vi "Chart.vi"() -> ()   [LabVIEW 2020]
uses:
  <userlib>/_NEVSTOP/Communicable State Machine(CSM)/AdvanceAPI/CSM - Revert Arguments-Safe String.vi
  <userlib>/_NEVSTOP/Communicable State Machine(CSM)/_Shared/Trim Single-line Text.vi
  <userlib>/_NEVSTOP/Communicable State Machine(CSM)/AdvanceAPI/CSM - Make String Arguments Safe.vi
  <userlib>/_NEVSTOP/Communicable State Machine(CSM)/AdvanceAPI/CSM - Break Down Multiple States String.vi
  <userlib>/_NEVSTOP/Communicable State Machine(CSM)/AdvanceAPI/CSM - Compact Multiple States.vi
  <userlib>/_NEVSTOP/Communicable State Machine(CSM)/AdvanceAPI/CSM - Keywords.vi
  <userlib>/_NEVSTOP/Communicable State Machine(CSM)/Communicable State Machine.lvlib
panel:
  out "Waveform Chart":dbl(graph)
  out "State History":string
  in  "Name (\"\" to Use UUID)":string="Event CSM"
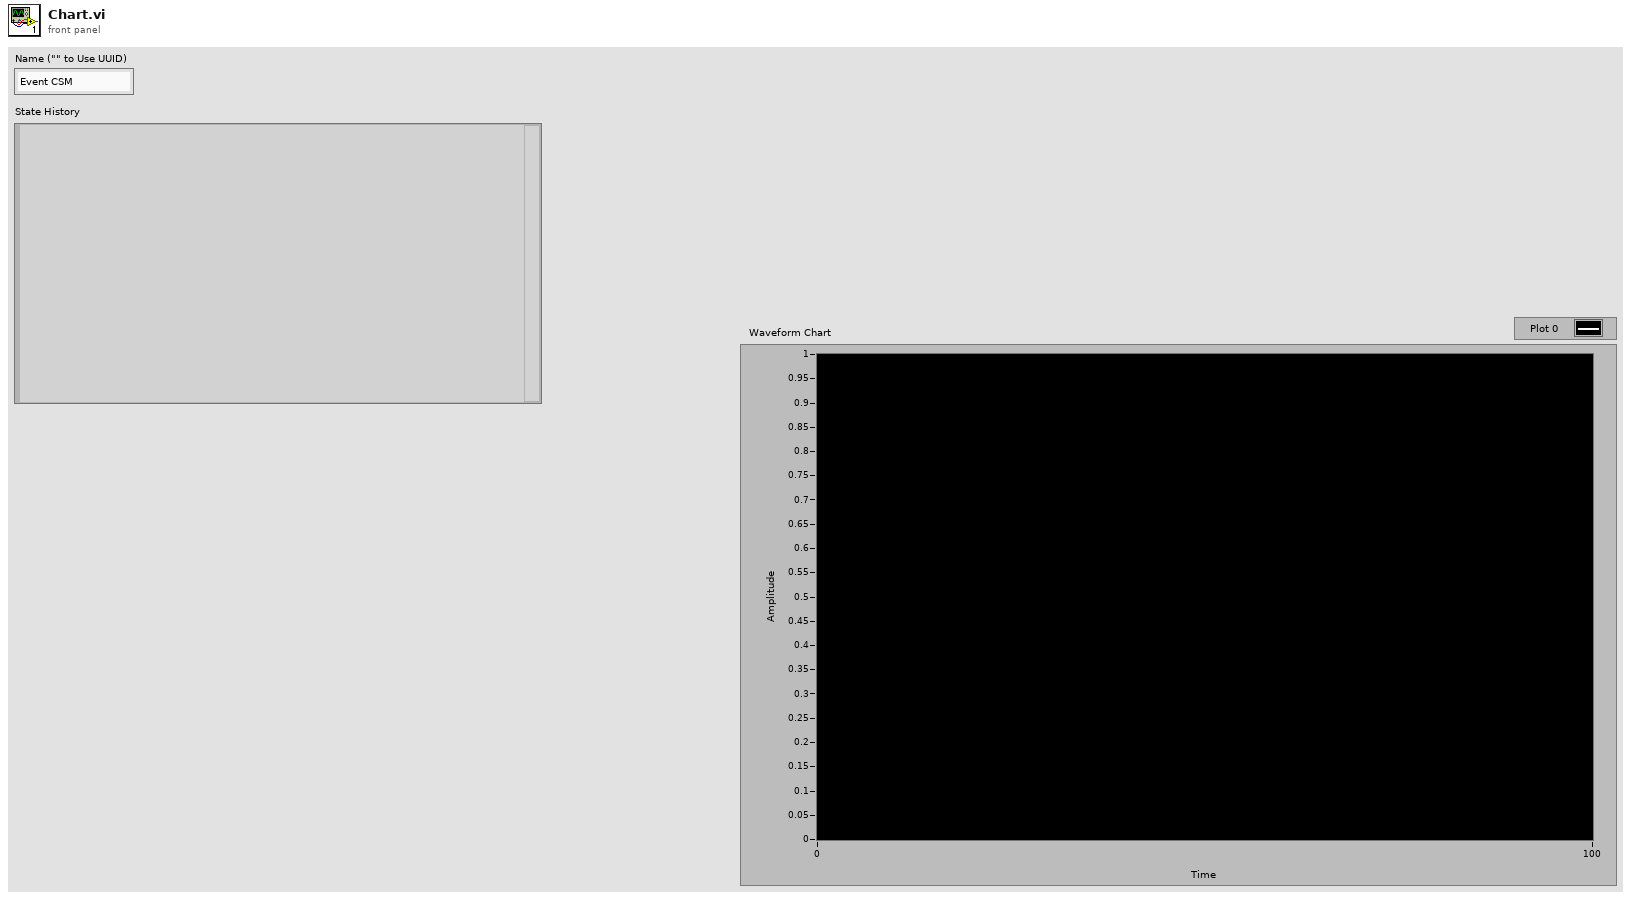
[diagram p1: front panel]
types:
  T1 = enum32{"Invalid", "Standard", "Closed", "Hidden", "Minimized", "Maximized"}
  T2 = enum32{"invalid app kind", "Development System", "Run Time System", "Student Edition", "Embedded LabVIEW", "Evaluation", "Custom"}
  T3 = typedef "Communicable State Machine.lvlib/_CSM_Response Source Message.ctl" = cluster{"‘State":string, "’Arguments":string, "’Error":errorcluster}
  T4 = cluster{"Current VI Reference":refnum<vi>, "Close Panel on Exit?":bool}
  T5 = cluster{"Core":cluster{"Current VI Reference":refnum<vi>, "Close Panel on Exit?":bool}, "Your Boolean data":bool, "Your string data":string}
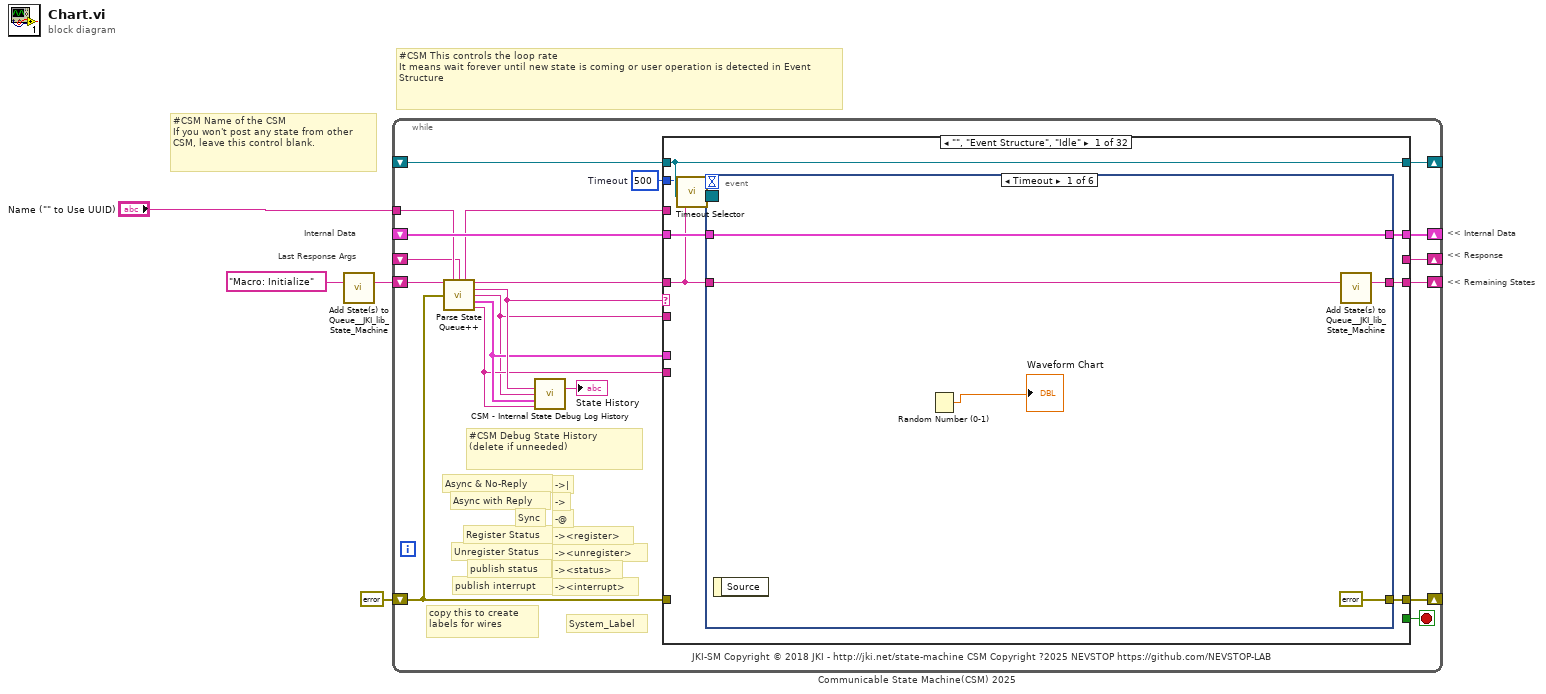
[diagram p0: block diagram]
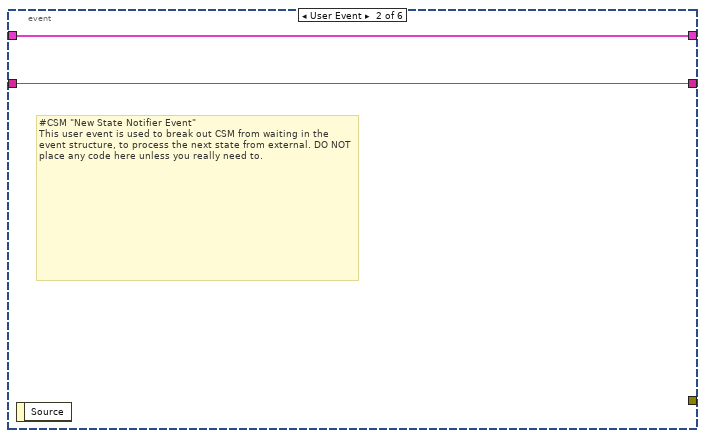
[diagram p2: hidden frame]
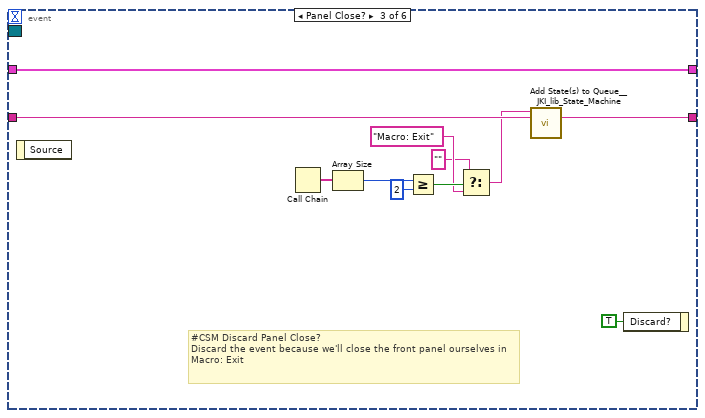
[diagram p3: hidden frame]
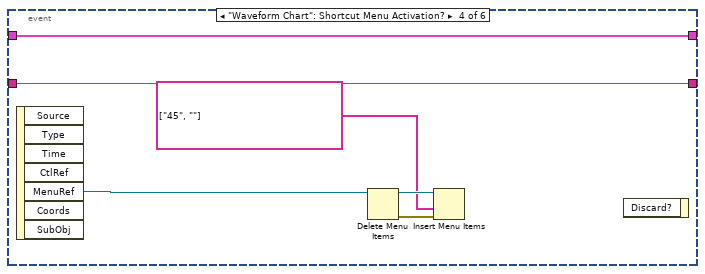
[diagram p4: hidden frame]
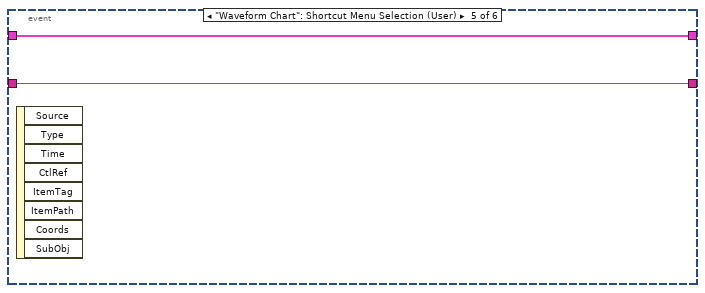
[diagram p5: hidden frame]
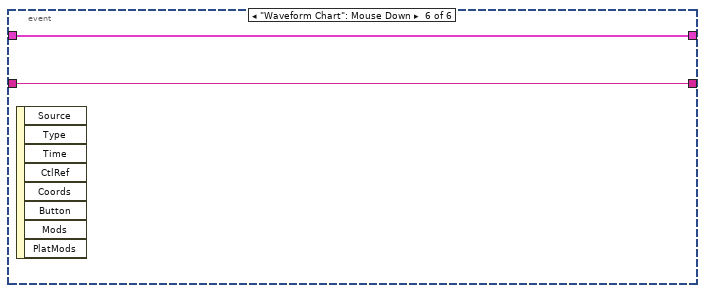
[diagram p6: hidden frame]
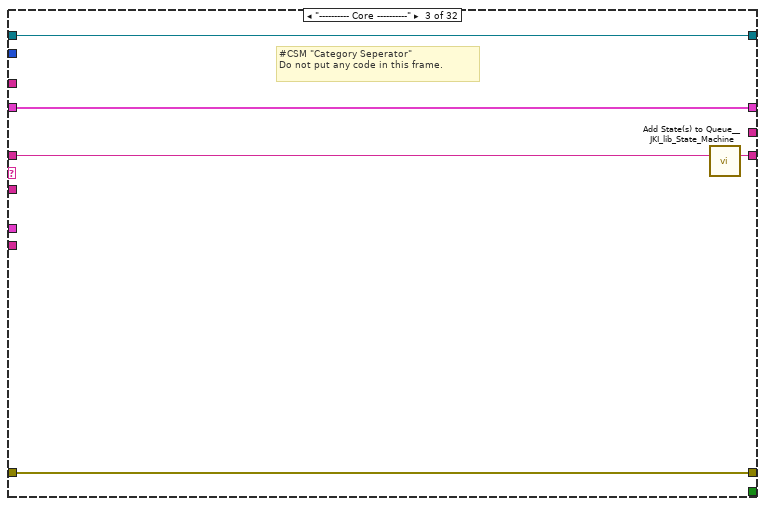
[diagram p8: hidden frame]
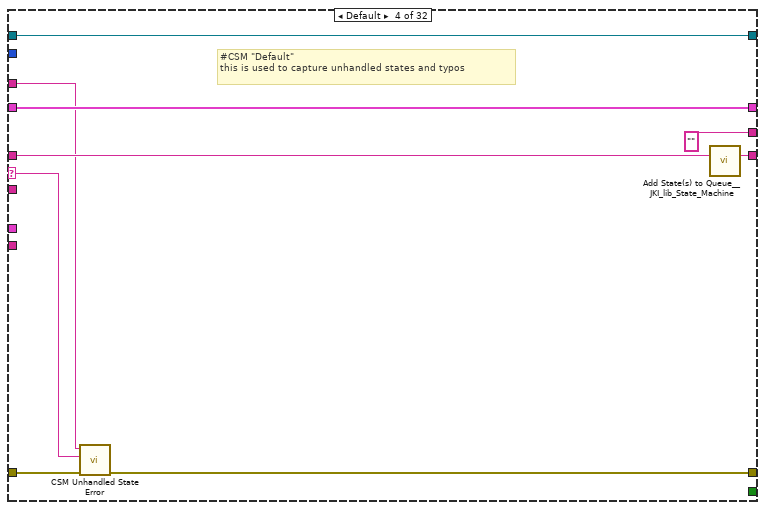
[diagram p9: hidden frame]
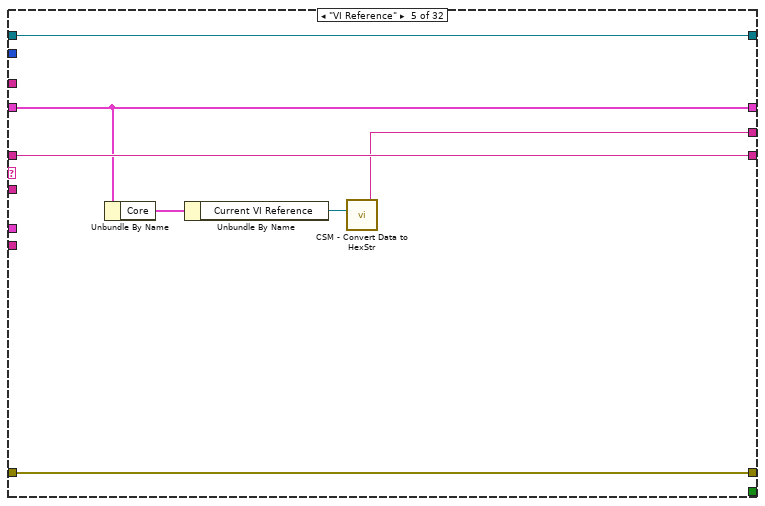
[diagram p10: hidden frame]
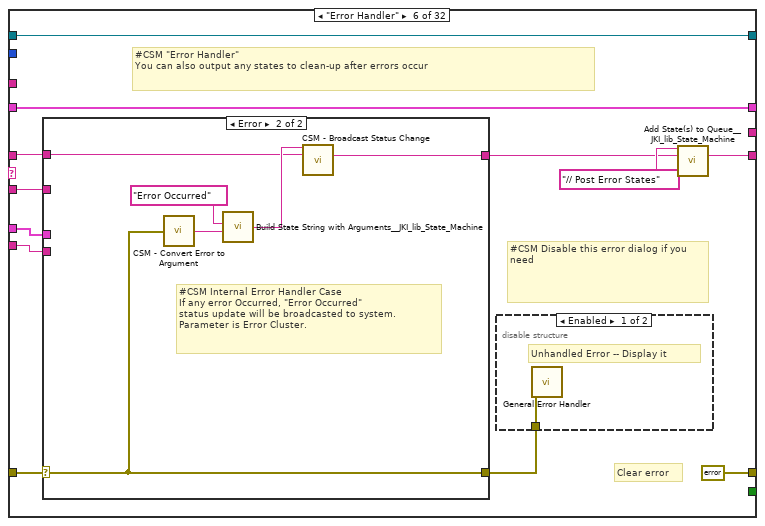
[diagram p11: hidden frame]
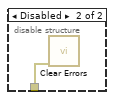
[diagram p12: hidden frame]
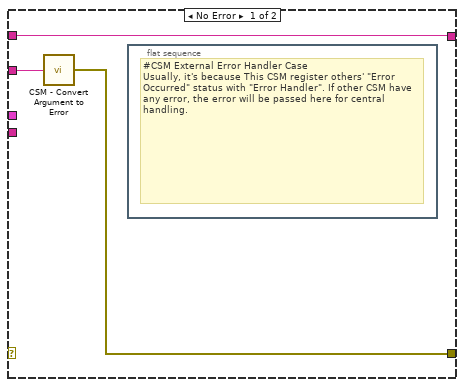
[diagram p13: hidden frame]
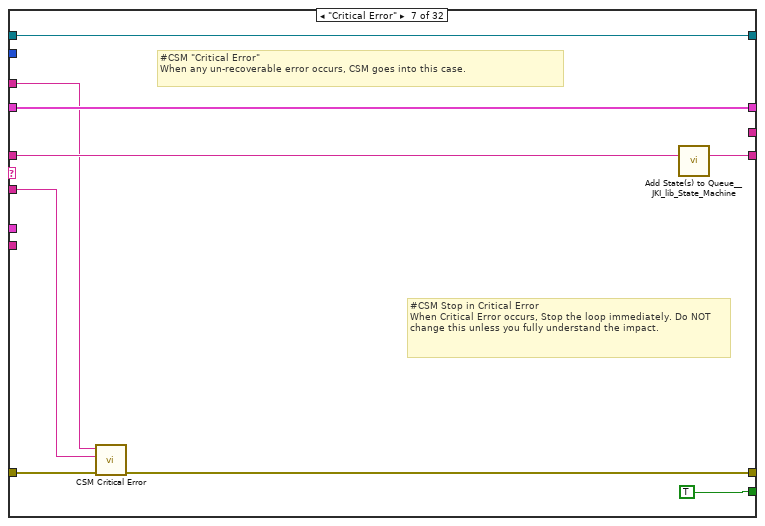
[diagram p14: hidden frame]
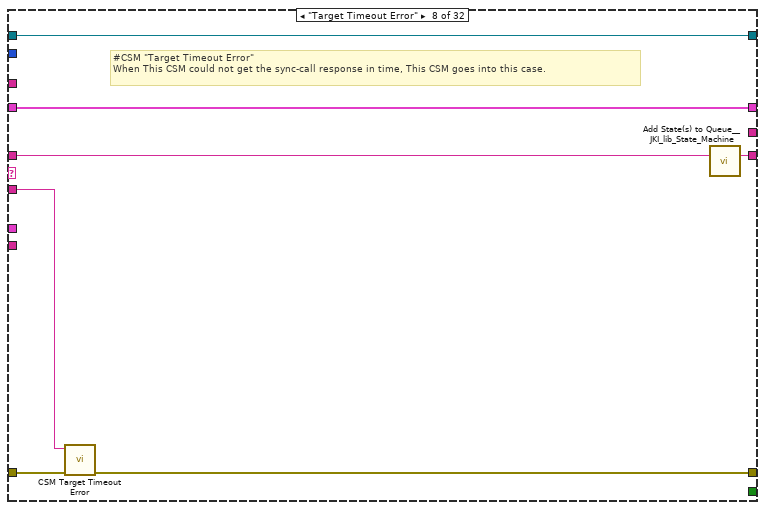
[diagram p15: hidden frame]
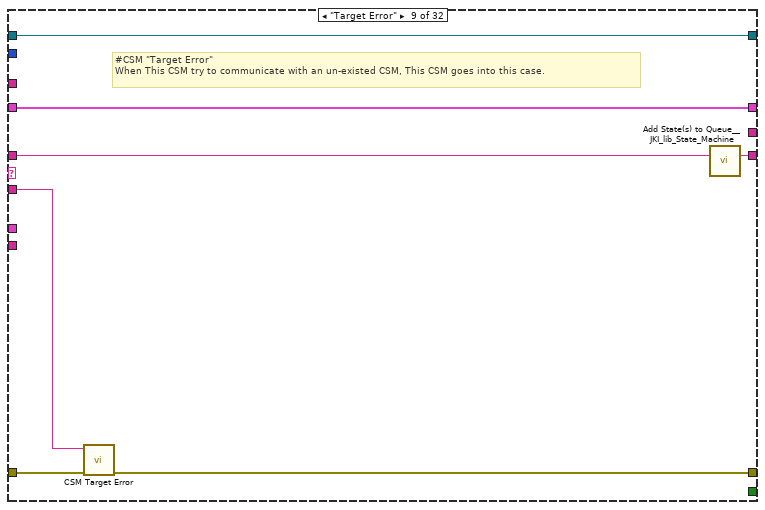
[diagram p16: hidden frame]
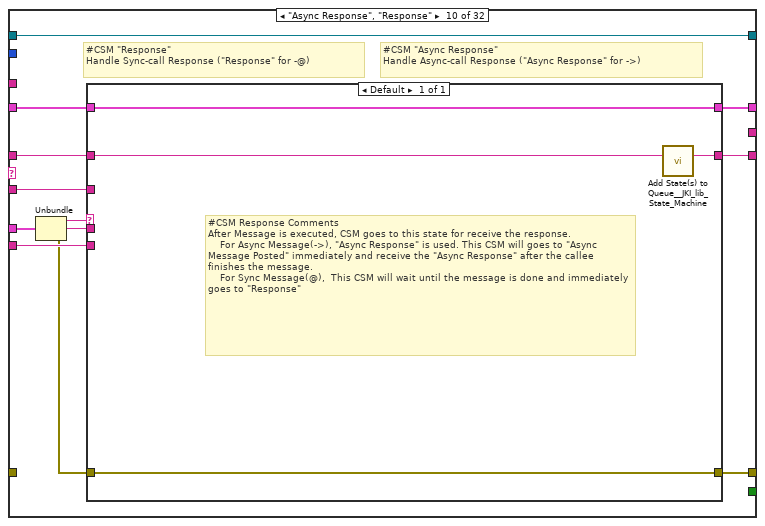
[diagram p17: hidden frame]
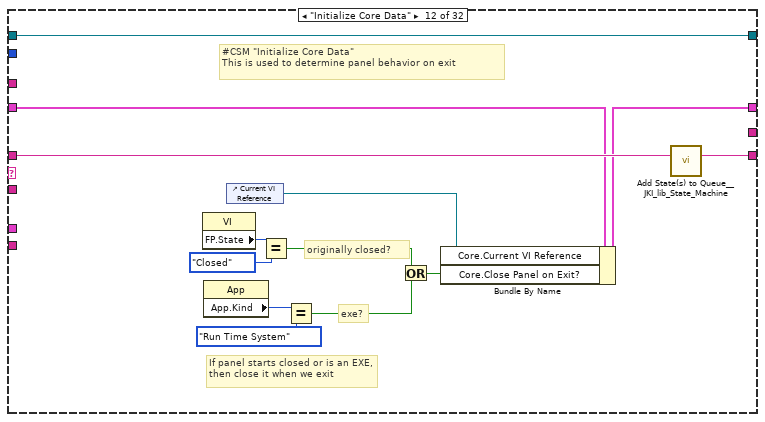
[diagram p19: hidden frame]
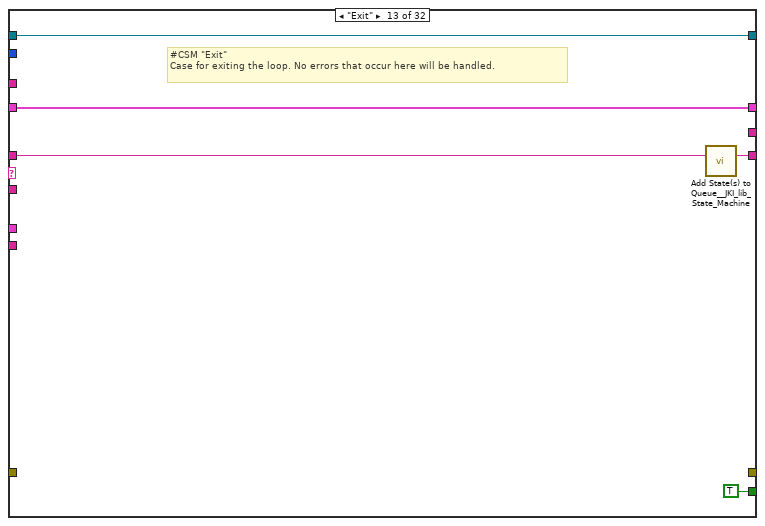
[diagram p20: hidden frame]
diagram:
  # "Last Response Args"
  # "Internal Data"
  # "<< Internal Data"
  # "<< Response"
  # "<< Remaining States"
  # "#CSM Name of the CSM\nIf you won't post any state from other CSM, leave this control blank."
  # "#CSM This controls the loop rate\nIt means wait forever until new state is coming or user operation is detected in Event Structure"
  n1 = call <vilib>:"Add State(s) to Queue__JKI_lib_State_Machine.vi"("State(s) in (\"\")"="Macro: Initialize" ("Init State(\"Macro: Initialize\")")) -> ("States Out"=w1:string)  [unwired: 14 in]
  n2 = while "Communicable State Machine(CSM) 2025" {
    shift-right: [w19] -> _
    shift-left: _ -> [w18]
    shift-right: [w22] -> _
    shift-left: errorcluster {"status"=FALSE, "code"=0, "source"=""} ("error out") -> [w16]
    shift-right: [w21] -> _
    shift-left: w1 -> [w23]
    tunnel: "Name (\"\" to Use UUID)" -> [w12]
    shift-right: [w15] -> _
    shift-left: _ -> [w7]
    shift-right: [w14] -> _
    shift-left: _ -> [w13]
    stop <- w20 stop-if-true
    w17 = 500  # Timeout
    # "#CSM Debug State History\n(delete if unneeded)"
    # "-><interrupt>"
    # "-><status>"
    # "-><unregister>"
    # "-><register>"
    # "-@"
    # "->"
    # "->|"
    # "publish interrupt"
    # "publish status"
    # "Unregister Status"
    # "Register Status"
    # "Sync"
    # "Async with Reply"
    # "Async & No-Reply"
    # "copy this to create labels for wires"
    # "System_Label"
    # "JKI-SM Copyright © 2018 JKI - http://jki.net/state-machine CSM Copyright ?2025 NEVSTOP https://github.com/NEVSTOP-LAB"
    n3 = call <userlib>:"Parse State Queue++.vi"("State Queue"=w23, "Name (\"\" to Use UUID)"=w12, "Response Arguments"=w7, "Previous Error"=w16) -> ("Name Used"=w8:string, "Remaining States"=w24:string, "Current State"=w11:string, "Arguments"=w6:string, "Additional Information"=w10:T3, "Source CSM"=w9:string)  [unwired: 6 in]
    n4 = call <userlib>:"CSM - Internal State Debug Log History.vi"("State"=w11, "Arguments (\"\")"=w6, ">> Response Source Message >>"=w10, "Source (\"\")"=w9) -> ("Debug Log"=→"State History":string)  [unwired: 11 in]
    n5 = case shown="\"\", \"Event Structure\", \"Idle\"" w11 {
      selector: w11 -> [_ _ _ w71 _ _ _ _ _ _ _ _ _ _ _ _ _ _ _ _ _ _ _ _ _ _ _ _ _ _ _ _]
      tunnel: w24 -> [w25 w63 w68 w77 w83 w89 w115 w123 w130 w140 w149 w162 w167 w171 w178 w184 w188 w195 w199 w203 w207 w213 w224 w288 w293 w304 w307 w311 w314 w318 w322 w326]
      tunnel: w6 -> [_ _ _ _ _ w87 w111 w118 w126 w134 _ _ _ _ _ _ _ _ _ _ _ w209 w219 _ _ _ _ _ _ _ _ _]
      tunnel: w18 -> [w31 w62 w65 w75 w82 w95 w116 w121 w128 w138 w148 w156 w165 w169 _ w180 w186 w194 w198 w201 w205 w211 w221 w286 w291 w302 w306 w310 w313 w316 w320 w324]
      tunnel: [w30 _ w66 w69 w84 errorcluster {"status"=FALSE, "code"=0, "source"=""} ("error out") w108 w117 w124 w137 _ _ _ _ _ w181 _ w189 w197 _ _ w210 w222 _ _ _ _ _ _ _ _ _] -> w22
      tunnel: w16 -> [_ _ w66 w70 w84 w93 w109 w119 w125 _ _ _ _ _ _ _ _ _ _ _ _ _ _ _ _ _ _ _ _ _ _ _]
      tunnel: [w32 w63 w67 w76 w83 w91 w114 w122 w129 w141 w149 w161 w166 w170 w177 w183 w187 w195 w199 w202 w206 w212 w223 w287 w292 w303 w307 w311 w314 w317 w321 w325] -> w21
      tunnel: [_ _ _ _ _ _ TRUE _ _ _ _ _ TRUE _ _ _ _ _ _ _ _ _ _ _ _ _ _ _ _ _ _ _] -> w20
      tunnel: [w29 w62 w65 w75 w82 w95 w116 w121 w128 w139 w148 w160 w165 w169 w176 w180 w186 w194 w198 w201 w205 w211 w221 w286 w291 w302 w306 w310 w313 w316 w320 w324] -> w19
      tunnel: w17 -> [w27 _ _ _ _ _ _ _ _ _ _ _ _ _ _ _ _ _ _ _ _ _ _ _ _ _ _ _ _ _ _ _]
      tunnel: w9 -> [_ _ _ _ _ w86 _ _ _ w135 _ _ _ _ _ _ _ _ _ _ _ _ _ _ _ _ _ _ _ _ _ _]
      tunnel: w10 -> [_ _ _ _ _ w85 _ _ _ w136 _ _ _ _ _ _ _ _ _ _ _ _ _ _ _ _ _ _ _ _ _ _]
      tunnel: [_ _ _ "" w78 _ _ _ _ _ _ _ _ _ _ _ _ _ _ _ _ _ _ _ _ _ _ "API1 Response" _ _ _ _] -> w15
      tunnel: [w28 w61 w64 w73 w81 w94 w112 w120 w127 w142 w147 w150 w163 w168 w172 w179 w185 w193 w196 w200 w204 w208 w218 w285 w289 w295 w305 w309 w312 w315 w319 w323] -> w14
      tunnel: w13 -> [w28 w61 w64 w73 w81 w94 w112 w120 w127 w142 w147 w150 w163 w168 w172 w179 w185 _ w196 w200 w204 w208 w218 w285 w289 w295 w305 w309 w312 w315 w319 w323]
      tunnel: w8 -> [_ _ _ w72 _ _ w110 _ _ _ _ _ _ _ _ _ _ w192 _ _ _ _ _ _ _ _ _ _ _ _ _ _]
      frame "", "Event Structure", "Idle" {
        n6 = call <userlib>:"Timeout Selector.vi"("Remaining States"=w25, "Timeout Expected"=w27) -> ("Timeout"=w26:i32)  [unwired: 5 in]
        n7 = event shown="[0] Timeout" {
          selector: w28 -> [_ _ _ _ _ _]
          dyn-events: _ -> [_ _ _ _ _ _]
          timeout: w26 -> [_ _ _ _ _ _]
          tunnel: w25 -> [w37 w38 w50 w56 w58 w60]
          tunnel: [w36 w38 w49 w56 w58 w60] -> w32
          tunnel: w31 -> [w35 w39 w48 w55 w57 w59]
          tunnel: [errorcluster {"status"=FALSE, "code"=0, "source"=""} ("error out") _ _ _ _ _] -> w30
          tunnel: [w35 w39 w48 w55 w57 w59] -> w29
          event Timeout {
            n8 = event-data() -> ()  [unwired: 1 in, 1 out]
            n9 = Random Number (0-1)() -> (number: 0 to 1=→"Waveform Chart":dbl)
            n10 = call <vilib>:"Add State(s) to Queue__JKI_lib_State_Machine.vi"("State(s) in (\"\")"=w37) -> ("States Out"=w36:string)  [unwired: 14 in]
          }
          event User Event {
            # "#CSM \"New State Notifier Event\"\nThis user event is used to break out CSM from waiting in the event structure, to process the next state from external. DO NOT place any code here unless you really need to."
            n11 = event-data() -> ()  [unwired: 1 in, 1 out]
          }
          event Panel Close? {
            # "#CSM Discard Panel Close?\nDiscard the event because we'll close the front panel ourselves in Macro: Exit"
            n12 = event-data() -> ()  [unwired: 1 in, 1 out]
            n13 = Call Chain() -> (call chain=w40:string[])
            n14 = Array Size(array=w40) -> (size(s)=w46:i32)
            n15 = Greater Or Equal?(x=w46, y=2) -> (x >= y?=w44:bool)
            n16 = Select(t="", s=w44, f="Macro: Exit") -> (s? t:f=w41:string)
            n17 = call <vilib>:"Add State(s) to Queue__JKI_lib_State_Machine.vi"("State(s) in Front (\"\")"=w41, "State(s) in (\"\")"=w50) -> ("States Out"=w49:string)  [unwired: 13 in]
            n18 = event-data("Discard?"=TRUE) -> ()  [unwired: 1 in, 1 out]
          }
          event "Waveform Chart": Shortcut Menu Activation? {
            n19 = event-data() -> ("MenuRef"=w51:refnum<k9>)  [unwired: 1 in, 6 out]
            n20 = Delete Menu Items(9:w51) -> (0:w54:errorcluster, 3:w53:refnum<k9>)  [unwired: 3 in]
            n21 = Insert Menu Items(6:w54, 7:string[] ["45", ""] ("item names"), 9:w53) -> ()  [unwired: 3 in, 3 out]
            n22 = event-data() -> ()  [unwired: 2 in, 1 out]
          }
          event "Waveform Chart": Shortcut Menu Selection (User) {
            n23 = event-data() -> ()  [unwired: 1 in, 8 out]
          }
          event "Waveform Chart": Mouse Down {
            n24 = event-data() -> ()  [unwired: 1 in, 8 out]
          }
        }
      }
      frame "CSM Documentation" {
        # "#CSM State Syntax\n\n// Comment line, all text to the right of “//” will be ignored\n// Local Message Example\nDoSth: DoA >> Arguments\n\n// Sync Call Example\nAPI: xxxx >> Arguments -@ TargetModule\n\n// Async Call Example\nAPI: xxxx >> Arguments -> TargetModule\n\n// Async Call without Reply Example\nAPI: xxxx >> Arguments ->| TargetModule\n\n// Broadcast normal status:\nStatus >> StatusArguments  -><status>\n\n// Broadcast Interrupt status:\nInterrupt >> StatusArguments  -><interrupt>\n\n// Register Source Module's status to Handler Module\nStatus@Source Module >> Handler Module@Handler Module -><register>\n\n// Unegister Source Module's status\nStatus@Source Module >> Handler Module -><unregister>"
        # "#CSM README FIRST\n\nCommunicable State Machine(CSM) is a LabVIEW application framework that builds upon JKI State Machine(JKISM). It follows the pattern of JKISM and extends the keywords to describe message communication between modules, including concepts such as Sync-Message, Async-Message, Subscription/Unsubscription of status - essential elements for creating reusable code modules. For more information, please visit the CSM wiki: https://nevstop-lab.github.io/CSM-Wiki/\n\nFor instructions on JKI State Machine, visit: \n    http://jki.net/state-machine/\nFor information about CSM, visit: \n    https://github.com/NEVSTOP-LAB"
        # "#CSM \"Documentation\"\nCase for holding CSM Documenation"
      }
      frame "---------- Core ----------" {
        # "#CSM \"Category Seperator\"\nDo not put any code in this frame."
        n25 = call <vilib>:"Add State(s) to Queue__JKI_lib_State_Machine.vi"("State(s) in (\"\")"=w68) -> ("States Out"=w67:string)  [unwired: 14 in]
      }
      frame Default {
        # "#CSM \"Default\"\nthis is used to capture unhandled states and typos"
        n26 = call <userlib>:"CSM Unhandled State Error.vi"("error in (no error)"=w70, "Undefined State"=w71, "CSM Name"=w72) -> ("error out"=w69:errorcluster)  [unwired: 8 in]
        n27 = call <vilib>:"Add State(s) to Queue__JKI_lib_State_Machine.vi"("State(s) in (\"\")"=w77) -> ("States Out"=w76:string)  [unwired: 14 in]
      }
      frame "VI Reference" {
        n28 = Unbundle By Name(w82) -> ("Core"=w80:T4)
        n29 = Unbundle By Name(w80) -> ("Current VI Reference"=w79:refnum<vi>)
        n30 = call <userlib>:"CSM - Convert Data to HexStr.vi"("Variant"=w79) -> ("HEX String (0-9,A-F)"=w78:string)  [unwired: 8 in]
      }
      frame "Error Handler" {
        # "#CSM Disable this error dialog if you need"
        # "#CSM \"Error Handler\"\nYou can also output any states to clean-up after errors occur"
        # "Clear error"
        n31 = case shown="Error" w93 {
          selector: w93 -> [_ w102]
          tunnel: [w100 w104] -> w90
          tunnel: w89 -> [w100 w103]
          tunnel: [w99 w102] -> w88
          tunnel: w87 -> [w101 _]
          tunnel: w86 -> [_ _]
          tunnel: w85 -> [_ _]
          frame No Error {
            n32 = call <userlib>:"CSM - Convert Argument to Error.vi"("Argument"=w101) -> ("Error"=w99:errorcluster)  [unwired: 4 in]
            n33 = flat-sequence {
              frame #0 {
                # "#CSM External Error Handler Case\nUsually, it's because This CSM register others' \"Error Occurred\" status with \"Error Handler\". If other CSM have any error, the error will be passed here for central handling."
              }
            }
          }
          frame Error {
            # "#CSM Internal Error Handler Case \nIf any error Occurred, \"Error Occurred\" \nstatus update will be broadcasted to system.\nParameter is Error Cluster."
            n34 = call <userlib>:"CSM - Convert Error to Argument.vi"("Error"=w102) -> ("Argument"=w106:string)  [unwired: 4 in]
            n35 = call <vilib>:"Build State String with Arguments__JKI_lib_State_Machine.vi"("Arguments (\"\")"=w106, "State"="Error Occurred" ("Status with Arguments")) -> ("State with Arguments"=w105:string)  [unwired: 4 in]
            n36 = call <userlib>:"CSM - Broadcast Status Change.vi"("Status With Arguments"=w105, "State Queue"=w103) -> ("Remaining States"=w104:string)  [unwired: 13 in]
          }
        }
        n37 = disable-structure shown="Enabled" {
          disable-tunnel: w88 -> [w97 w98]
          frame Enabled {
            # "Unhandled Error -- Display it"
            n38 = call <vilib>:"General Error Handler.vi"("error in (no error)"=w97) -> ()  [unwired: 10 in, 5 out]
          }
          frame Disabled {
            n39 = call <vilib>:"Clear Errors.vi"("error in (no error)"=w98) -> ()  [unwired: 5 in, 2 out]
          }
        }
        n40 = call <vilib>:"Add State(s) to Queue__JKI_lib_State_Machine.vi"("State(s) in Front (\"\")"="// Post Error States", "State(s) in (\"\")"=w90) -> ("States Out"=w91:string)  [unwired: 13 in]
      }
      frame "Critical Error" {
        # "#CSM \"Critical Error\"\nWhen any un-recoverable error occurs, CSM goes into this case."
        # "#CSM Stop in Critical Error\nWhen Critical Error occurs, Stop the loop immediately. Do NOT change this unless you fully understand the impact."
        n41 = call <userlib>:"CSM Critical Error.vi"("error in (no error)"=w109, "Arugments (As Reason)"=w111, "CSM Name"=w110) -> ("error out"=w108:errorcluster)  [unwired: 8 in]
        n42 = call <vilib>:"Add State(s) to Queue__JKI_lib_State_Machine.vi"("State(s) in (\"\")"=w115) -> ("States Out"=w114:string)  [unwired: 14 in]
      }
      frame "Target Timeout Error" {
        # "#CSM \"Target Timeout Error\"\nWhen This CSM could not get the sync-call response in time, This CSM goes into this case."
        n43 = call <userlib>:"CSM Target Timeout Error.vi"("error in (no error)"=w119, "Arguments (As CSM Name)"=w118) -> ("error out"=w117:errorcluster)  [unwired: 9 in]
        n44 = call <vilib>:"Add State(s) to Queue__JKI_lib_State_Machine.vi"("State(s) in (\"\")"=w123) -> ("States Out"=w122:string)  [unwired: 14 in]
      }
      frame "Target Error" {
        # "#CSM \"Target Error\"\nWhen This CSM try to communicate with an un-existed CSM, This CSM goes into this case."
        n45 = call <userlib>:"CSM Target Error.vi"("error in (no error)"=w125, "Arguments (As CSM Name)"=w126) -> ("error out"=w124:errorcluster)  [unwired: 9 in]
        n46 = call <vilib>:"Add State(s) to Queue__JKI_lib_State_Machine.vi"("State(s) in (\"\")"=w130) -> ("States Out"=w129:string)  [unwired: 14 in]
      }
      frame "Async Response", "Response" {
        # "#CSM \"Async Response\"\nHandle Async-call Response (\"Async Response\" for ->)"
        # "#CSM \"Response\"\nHandle Sync-call Response (\"Response\" for -@)"
        n47 = Unbundle(w136) -> ("‘State"=w133:string, "’Arguments"=w132:string, "’Error"=w131:errorcluster)
        n48 = case shown="Default" w133 {
          tunnel: [w143] -> w141
          tunnel: w140 -> [w144]
          tunnel: [w146] -> w139
          tunnel: w138 -> [w146]
          tunnel: [w145] -> w137
          tunnel: w131 -> [w145]
          tunnel: w135 -> [_]
          tunnel: w134 -> [_]
          tunnel: w132 -> [_]
          frame Default {
            # "#CSM Response Comments\nAfter Message is executed, CSM goes to this state for receive the response.\n    For Async Message(->), \"Async Response\" is used. This CSM will goes to \"Async Message Posted\" immediately and receive the \"Async Response\" after the callee finishes the message.\n    For Sync Message(@),  This CSM will wait until the message is done and immediately goes to \"Response\""
            n49 = call <vilib>:"Add State(s) to Queue__JKI_lib_State_Machine.vi"("State(s) in (\"\")"=w144) -> ("States Out"=w143:string)  [unwired: 14 in]
          }
        }
      }
      frame "Async Message Posted" {
        # "#CSM \"Async Message Posted\"\nAfter Async Message is posted (-> or ->| ), CSM goes to this state for post-action.\nYou can use Argument - State to tell which Async Message is called."
      }
      frame "Initialize Core Data" {
        # "#CSM \"Initialize Core Data\"\nThis is used to determine panel behavior on exit"
        # "originally closed?"
        # "exe?"
        # "If panel starts closed or is an EXE, then close it when we exit"
        n50 = property class="VI"() -> ("FP.State"=w153:T1)  [unwired: 2 in, 2 out]
        n51 = property class="App"() -> ("App.Kind"=w159:T2)  [unwired: 2 in, 2 out]
        n52 = control-ref of="Current VI Reference"() -> (w154:refnum<vi>)
        n53 = Equal?(x=w153, y=T1."Closed" ("Front Panel Window:State")) -> (x = y?=w151:bool)
        n54 = Equal?(x=w159, y=T2."Run Time System" ("Application:Kind")) -> (x = y?=w157:bool)
        n55 = Or(x=w151, y=w157) -> (x .or. y?=w155:bool)
        n56 = Bundle By Name(cluster=w156, "Core.Current VI Reference"=w154, "Core.Close Panel on Exit?"=w155) -> (w160:T5)
        n57 = call <vilib>:"Add State(s) to Queue__JKI_lib_State_Machine.vi"("State(s) in (\"\")"=w162) -> ("States Out"=w161:string)  [unwired: 14 in]
      }
      frame "Exit" {
        # "#CSM \"Exit\"\nCase for exiting the loop. No errors that occur here will be handled."
        n58 = call <vilib>:"Add State(s) to Queue__JKI_lib_State_Machine.vi"("State(s) in (\"\")"=w167) -> ("States Out"=w166:string)  [unwired: 14 in]
      }
      frame "---------- Data ----------" {
        # "#CSM \"Category Seperator\"\nDo not put any code in this frame."
        n59 = call <vilib>:"Add State(s) to Queue__JKI_lib_State_Machine.vi"("State(s) in (\"\")"=w171) -> ("States Out"=w170:string)  [unwired: 14 in]
      }
      frame "Data: Initialize" {
        w173 = T4 {"Current VI Reference"=refnum, "Close Panel on Exit?"=FALSE}  # Core
        w175 = TRUE  # Your Boolean data
        w174 = ""  # Your string data
        # "#CSM  do not delete - used by framework"
        # "#CSM Expand Bundle to add new data elements to shift register data."
        # "#CSM Add new data here."
        # "#CSM Data names and types of shift register data are defined by this bundle."
        # "#CSM \"Data: Initialize\"\nInitialize the shift-register data, here.\n(data names are defined by what you wire into the bundle function)"
        n60 = Bundle("Core"=w173, "Your Boolean data"=w175, "Your string data"=w174) -> (w176:T5)  [unwired: 1 in]
        n61 = call <vilib>:"Add State(s) to Queue__JKI_lib_State_Machine.vi"("State(s) in (\"\")"=w178) -> ("States Out"=w177:string)  [unwired: 14 in]
      }
      frame "Data: Cleanup" {
        # "#CSM \"Data: Cleanup\"\nCleanup any data and references, here.\n(this is called automatically, by the Macro: Exit)"
        n62 = Unbundle By Name(w180) -> ("Core.Current VI Reference"=w182:refnum<vi>)
        n63 = Close Reference(reference=w182) -> (error out=w181:errorcluster)  [unwired: 1 in]
        n64 = call <vilib>:"Add State(s) to Queue__JKI_lib_State_Machine.vi"("State(s) in (\"\")"=w184) -> ("States Out"=w183:string)  [unwired: 14 in]
      }
      frame "---------- Events ----------" {
        # "#CSM \"Category Seperator\"\nDo not put any code in this frame."
        n65 = call <vilib>:"Add State(s) to Queue__JKI_lib_State_Machine.vi"("State(s) in (\"\")"=w188) -> ("States Out"=w187:string)  [unwired: 14 in]
      }
      frame "Events: Register" {
        # "#CSM \"Events: Register\"\nRegister user event. New Message Event is registered to break CSM waiting in event structure by default."
        # "#CSM Register New Message Event\nRegister message event to break Waiting in Event structure."
        n66 = call <userlib>:"CSM - Get New State Notifier Event.vi"("Name (\"\" to Use UUID)"=w192) -> ("error out"=w190:errorcluster, "New State Notifier Event"=w191:refnum<user-event>)  [unwired: 9 in]
        n67 = register-events(error in=w190, w191) -> (reference out=w193:refnum<event-registration>, error out=w189:errorcluster)  [unwired: 1 in]
      }
      frame "Events: Unregister" {
        # "#CSM \"Events: Unregister\"\nUnregister user event."
        n68 = Unregister For Events(event registration refnum=w196) -> (error out=w197:errorcluster)  [unwired: 1 in]
      }
      frame "---------- UI ----------" {
        # "#CSM \"Category Seperator\"\nDo not put any code in this frame."
        n69 = call <vilib>:"Add State(s) to Queue__JKI_lib_State_Machine.vi"("State(s) in (\"\")"=w203) -> ("States Out"=w202:string)  [unwired: 14 in]
      }
      frame "UI: Initialize" {
        # "#CSM \"UI: Initialize\"\nInitialize the User Interface, here.\n(this is called automatically, by the Macro: Init)"
        n70 = call <vilib>:"Add State(s) to Queue__JKI_lib_State_Machine.vi"("State(s) in (\"\")"=w207) -> ("States Out"=w206:string)  [unwired: 14 in]
      }
      frame "UI: Cursor Set" {
        # "Argument"
        # "#CSM \"UI: Cursor Set\"\nSet and Unset Cursor Busy.\n(Usage: \"UI: Cursor Set >> Busy|Idle\")"
        n71 = disable-structure shown="TARGET_TYPE!=Windows" {
          disable-tunnel: [w215 _] -> w210
          disable-tunnel: w209 -> [w214 _]
          frame condition #0 (active) {
            n72 = case shown="\"Idle\", Default" w214 {
              tunnel: [w216 w217] -> w215
              frame "Idle", Default {
                n73 = call <vilib>:"Unset Busy.vi"() -> ("error out"=w216:errorcluster)  [unwired: 11 in]
              }
              frame "Busy" {
                n74 = call <vilib>:"Set Busy.vi"() -> ("error out"=w217:errorcluster)  [unwired: 10 in, 1 out]
              }
            }
          }
          frame condition #1 {
          }
        }
        n75 = call <vilib>:"Add State(s) to Queue__JKI_lib_State_Machine.vi"("State(s) in (\"\")"=w213) -> ("States Out"=w212:string)  [unwired: 14 in]
      }
      frame "UI: Front Panel State" {
        # "Argument"
        # "#CSM \"UI: Front Panel State\"\nSet Front Panel Open or Closed\n(Usage: \"UI: Front Panel State >> Open|Close\")"
        n76 = Unbundle By Name(w221) -> ("Core.Current VI Reference"=w220:refnum<vi>)
        n77 = case shown="\"Open\", \"Standard\", Default" w219 {
          tunnel: [w231 w244 w255 w267 w279] -> w222
          tunnel: w220 -> [w230 w242 w254 w266 w278]
          frame "Open", "Standard", Default {
            w225 = T1."Standard" ("State")
            n78 = property class="VI"(reference=w230) -> (reference out=w228:refnum<vi>, error out=w229:errorcluster, "FP.State"=w227:T1)  [unwired: 1 in]
            n79 = Not Equal?(x=w227, y=w225) -> (x != y?=w226:bool)
            n80 = case shown="True" w226 {
              tunnel: [w235 w237] -> w231
              tunnel: w229 -> [w234 w237]
              tunnel: w228 -> [w233 _]
              tunnel: w225 -> [w232 _]
              frame True {
                n81 = invoke class="VI" method="FP.Open"(reference=w233, error in=w234, "Activate"=TRUE, "State"=w232) -> (error out=w235:errorcluster)  [unwired: 1 in, 4 out]
              }
              frame False {
              }
            }
          }
          frame "Close", "Closed" {
            n82 = property class="VI"(reference=w242) -> (reference out=w241:refnum<vi>, error out=w243:errorcluster, "FP.State"=w239:T1)  [unwired: 1 in]
            n83 = Not Equal?(x=w239, y=T1."Closed" ("Front Panel Window:State")) -> (x != y?=w238:bool)
            n84 = case shown="True" w238 {
              tunnel: [w245 w248] -> w244
              tunnel: w243 -> [w245 w247]
              tunnel: w241 -> [_ w246]
              frame False {
              }
              frame True {
                n85 = invoke class="VI" method="FP.Close"(reference=w246, error in=w247) -> (error out=w248:errorcluster)  [unwired: 1 in, 2 out]
              }
            }
          }
          frame "Hidden", "Hide" {
            w249 = T1."Hidden" ("State")
            n86 = property class="VI"(reference=w254) -> (reference out=w252:refnum<vi>, error out=w253:errorcluster, "FP.State"=w251:T1)  [unwired: 1 in]
            n87 = Not Equal?(x=w251, y=w249) -> (x != y?=w250:bool)
            n88 = case shown="True" w250 {
              tunnel: [w259 w260] -> w255
              tunnel: w253 -> [w258 w260]
              tunnel: w252 -> [w257 _]
              tunnel: w249 -> [w256 _]
              frame True {
                n89 = invoke class="VI" method="FP.Open"(reference=w257, error in=w258, "State"=w256) -> (error out=w259:errorcluster)  [unwired: 2 in, 4 out]
              }
              frame False {
              }
            }
          }
          frame "Minimize", "Minimized" {
            w261 = T1."Minimized" ("State")
            n90 = property class="VI"(reference=w266) -> (reference out=w264:refnum<vi>, error out=w265:errorcluster, "FP.State"=w263:T1)  [unwired: 1 in]
            n91 = Not Equal?(x=w263, y=w261) -> (x != y?=w262:bool)
            n92 = case shown="False" w262 {
              tunnel: [w271 w272] -> w267
              tunnel: w265 -> [w270 w272]
              tunnel: w264 -> [w269 _]
              tunnel: w261 -> [w268 _]
              frame True {
                n93 = invoke class="VI" method="FP.Open"(reference=w269, error in=w270, "State"=w268) -> (error out=w271:errorcluster)  [unwired: 2 in, 4 out]
              }
              frame False {
              }
            }
          }
          frame "Maximize", "Maximized" {
            w273 = T1."Maximized" ("State")
            n94 = property class="VI"(reference=w278) -> (reference out=w276:refnum<vi>, error out=w277:errorcluster, "FP.State"=w275:T1)  [unwired: 1 in]
            n95 = Not Equal?(x=w275, y=w273) -> (x != y?=w274:bool)
            n96 = case shown="True" w274 {
              tunnel: [w283 w284] -> w279
              tunnel: w277 -> [w282 w284]
              tunnel: w276 -> [w281 _]
              tunnel: w273 -> [w280 _]
              frame True {
                n97 = invoke class="VI" method="FP.Open"(reference=w281, error in=w282, "State"=w280) -> (error out=w283:errorcluster)  [unwired: 2 in, 4 out]
              }
              frame False {
              }
            }
          }
        }
        n98 = call <vilib>:"Add State(s) to Queue__JKI_lib_State_Machine.vi"("State(s) in (\"\")"=w224) -> ("States Out"=w223:string)  [unwired: 14 in]
      }
      frame "---------- Macro ----------" {
        # "#CSM \"Category Seperator\"\nDo not put any code in this frame."
        n99 = call <vilib>:"Add State(s) to Queue__JKI_lib_State_Machine.vi"("State(s) in (\"\")"=w288) -> ("States Out"=w287:string)  [unwired: 14 in]
      }
      frame "Macro: Initialize" {
        w290 = "Data: Initialize\nInitialize Core Data\nEvents: Register\nUI: Initialize\n//UI: Front Panel State >> Open"  # Data: Initialize Initialize Core Data Events: Register UI: Initialize //UI: Front Panel State >> Open
        # "#CSM \"Macro: Initialize\"\nInitialization Macro (This is called once, when the VI starts)"
        n100 = call <vilib>:"Add State(s) to Queue__JKI_lib_State_Machine.vi"("State(s) in Front (\"\")"=w290, "State(s) in (\"\")"=w293) -> ("States Out"=w292:string)  [unwired: 13 in]
      }
      frame "Macro: Exit" {
        # "#CSM \"Macro: Exit\"\nExit Macro (This is called once, when the VI exits)"
        n101 = Unbundle By Name(w302) -> ("Core.Close Panel on Exit?"=w301:bool)
        n102 = Select(t="UI: Front Panel State >> Close", s=w301, f="") -> (s? t:f=w298:string)
        n103 = call <vilib>:"Add State(s) to Queue__JKI_lib_State_Machine.vi"("State(s) in Front (\"\")"="//Exit Sub-Modules ", "State(s) in (\"\")"=w298, "State(s) at Back (\"\")"="Data: Cleanup\nEvents: Unregister\nExit") -> ("States Out"=w296:string)  [unwired: 12 in]
        n104 = call <vilib>:"Add State(s) to Queue__JKI_lib_State_Machine.vi"("State(s) in Front (\"\")"=w296, "State(s) in (\"\")"=w304) -> ("States Out"=w303:string)  [unwired: 13 in]
      }
      frame "---------- API ----------" {
        # "#CSM \"Category Seperator\"\nDo not put any code in this frame."
      }
      frame "API: API1" {
        # "#CSM >> Source CSM >>\nIf you need to tell who triggered this state , use this string. If it's this case itself, this string is \"\"."
        # "#CSM >> Arguments >>\nDeal with the parameter if any"
        # "#CSM Response\nConnect this to return the response of your API"
        # "#CSM API Example\nCopy/Rename this case for your own API"
      }
      frame "API: API2" {
        # "#CSM API Example\nCopy/Rename this case for your own API"
      }
      frame "---------- Action ----------" {
        # "#CSM \"Category Seperator\"\nDo not put any code in this frame."
        n105 = call <vilib>:"Add State(s) to Queue__JKI_lib_State_Machine.vi"("State(s) in (\"\")"=w318) -> ("States Out"=w317:string)  [unwired: 14 in]
      }
      frame "Action: action1" {
        # "#CSM \"Internal State\"\nThis category is used for holding internal states"
        n106 = call <vilib>:"Add State(s) to Queue__JKI_lib_State_Machine.vi"("State(s) in (\"\")"=w322) -> ("States Out"=w321:string)  [unwired: 14 in]
      }
      frame "Action: action2" {
        # "#CSM \"Internal State\"\nThis category is used for holding internal states"
        n107 = call <vilib>:"Add State(s) to Queue__JKI_lib_State_Machine.vi"("State(s) in (\"\")"=w326) -> ("States Out"=w325:string)  [unwired: 14 in]
      }
    }
  }
